vi "Acquisition next state logic_May contain upgrade.vi"(0 "Message Queues":T5, 5 "Acquired z-plane index":i32, 7 "Logging queue element":T1={"Imaging Protocol"=enum."Live Imaging", "Number of Trials"=0, "Frame Size"=512, "# Averaged frames"=0, "Dwell time (us)"=0.0, "Index of Z-plane"=0, "Timelapse?"=FALSE, "Logging process is active"=FALSE, "Speed logging enabled"=FALSE, "tdms file ref"=refnum, "path"=path "", "Trial Number"=0, "Expected # points acquired"=FALSE, "Manually stopped"=FALSE, "Last trial"=FALSE, "Ch0 data"=[], "Ch1 data"=[], "Ref Data"=[], "Ref Frame Time"=[], "Image Time"=[], "Continuous Time"=[], "Ref X Length"=0, "Ref Y Length"=0, "# Ref Averaged frames"=0, "Ref Dwell time (us)"=0.0, "Points acquired"={"Ch0 last trial"=0, "Ch1 last trial"=0, "All trials"=0}, "HW Timings File"=refnum} {"Ref Dwell time (us)" format="%#.6g"; "Frame Size" items=["100X100"=100, "128X128"=128, "200X200"=200, "256X256"=256, "512X512"=512, "1024x1024"=1024, "2048x2048"=2048]; "Dwell time (us)" format="%#.6g"}, 9 "Imaging Protocol":T2=enum."Live Imaging", 11 "error in":errorcluster) -> (6 "Index of next Z-plane to acquire":i32, 15 "error out":errorcluster)   [LabVIEW 2020]
uses:
  User Interface/Queue/Message Queue/Typedefs/All Message Queues.ctl
  User Interface/Queue/Message Queue/Typedefs/Message Cluster.ctl
  Typedefs/Logging queue element.ctl
  Typedefs/Imaging Protocols enum.ctl
  Typedefs/Frame Size.ctl
  Typedefs/Acquired points count.ctl
  Typedefs/Read Write Enum.ctl
  Global Variables/General Globals.vi
  Typedefs/Top level VI states.ctl
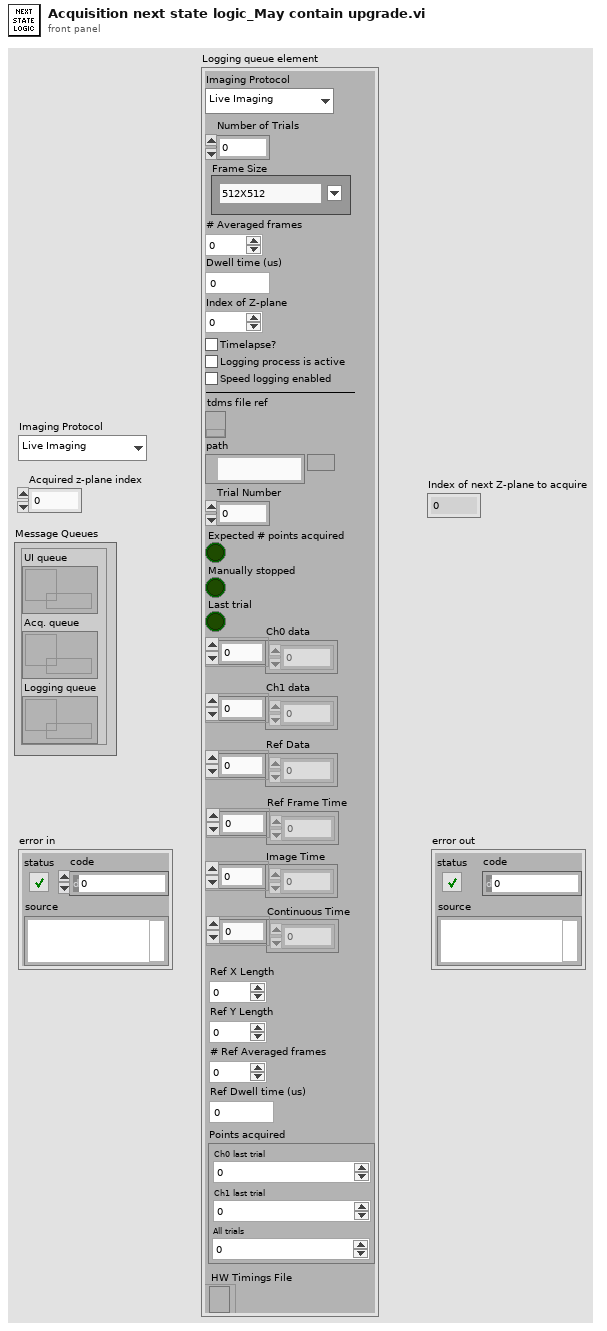
[diagram p1: front panel]
types:
  T1 = typedef "Logging queue element.ctl" = cluster{"Imaging Protocol":T2, "Number of Trials":u16, "Frame Size":T3, "# Averaged frames":u16, "Dwell time (us)":dbl, "Index of Z-plane":i32, "Timelapse?":bool, "Logging process is active":bool, "Speed logging enabled":bool, "tdms file ref":refnum<k34>, "path":path, "Trial Number":i32, "Expected # points acquired":bool, "Manually stopped":bool, "Last trial":bool, "Ch0 data":u32[], "Ch1 data":u32[], "Ref Data":u32[], "Ref Frame Time":u64[], "Image Time":u64[], "Continuous Time":u64[], "Ref X Length":u16, "Ref Y Length":u16, "# Ref Averaged frames":u16, "Ref Dwell time (us)":dbl, "Points acquired":T4, "HW Timings File":refnum<file>}
  T2 = typedef "Imaging Protocols enum.ctl" = enum16{"AOL Z-Stack", "Motor Z Stack", "Functional Acquisition", "Single Plane Acquisition", "Volume Acquisition", "Live Imaging", "Live Plane Imaging", "Live Volume Imaging"}
  T3 = typedef "Frame Size.ctl" = u16
  T4 = typedef "Acquired points count.ctl" = cluster{"Ch0 last trial":u64, "Ch1 last trial":u64, "All trials":u64}
  T5 = typedef "All Message Queues.ctl" = cluster{"UI queue":refnum<queue>, "Acq. queue":refnum<queue>, "Logging queue":refnum<queue>}
  T6 = typedef "Read Write Enum.ctl" = enum16{"Read", "Write"}
  T7 = typedef "Top level VI states.ctl" = enum16{"None", "Initialise UI", "<STACK PROTOCOL STATES>", "AOL Zstack-START", "AOL Zstack-STOP", "Motor Zstack-START", "Motor Zstack-STOP", "<ACQUISITION PROTOCOL STATES> ", "Functional Acquisition-START", "Functional Acquisition-STOP", "Single Plane Acquisition-START", "Single Plane Acquisition-STOP", "Volume Acquisition-START", "Volume Acquisition-STOP", "<LIVE IMAGING PROTOCOL STATES>", "Live Imaging-START", "Live Imaging-STOP", "Live Plane Imaging-START", "Live Plane Imaging-STOP", "Live Volume Imaging-START", "Live Volume Imaging-STOP", "<MOVEMENT CORRECTION PROTOCOL STATES>", "EXIT"}
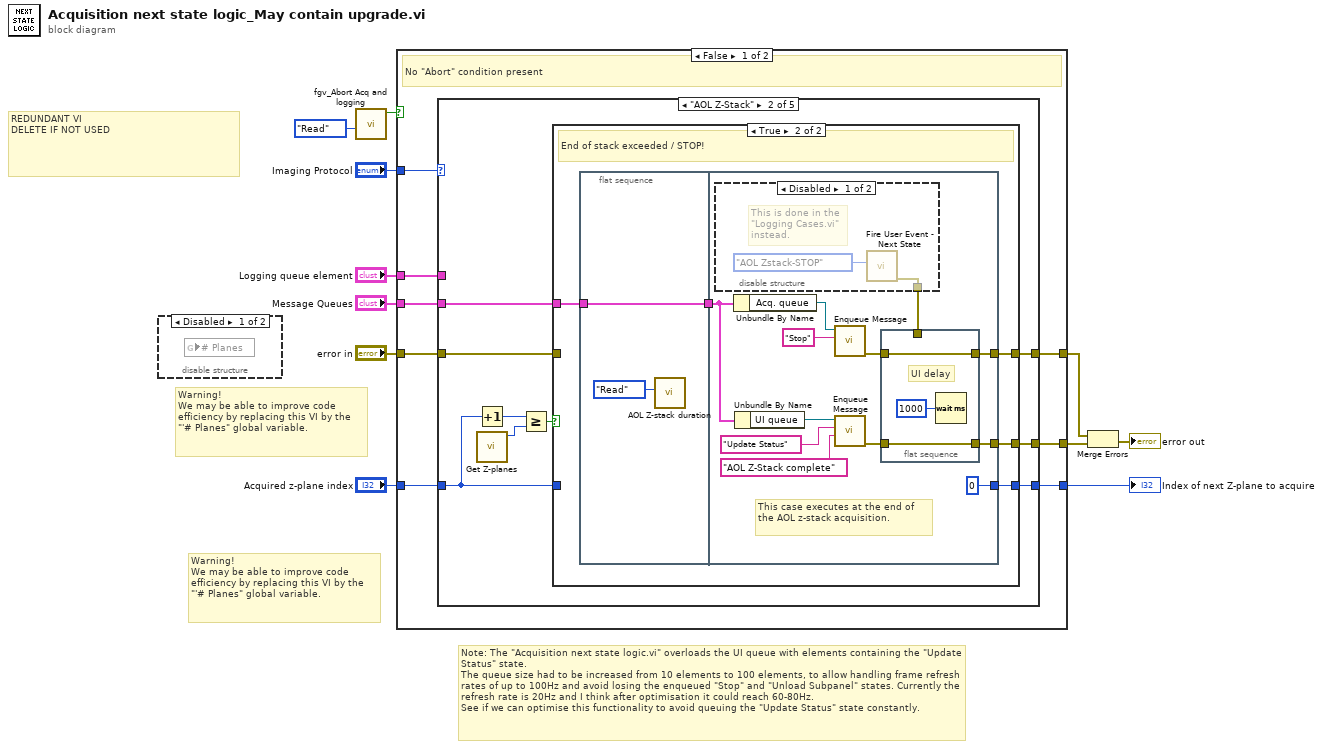
[diagram p0: block diagram]
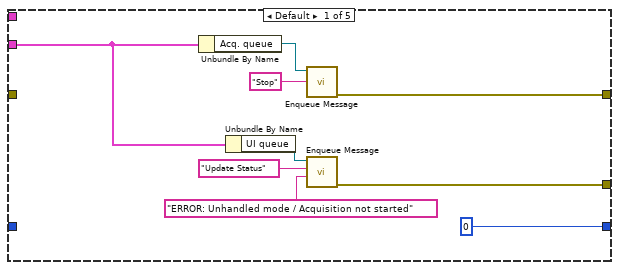
[diagram p3: hidden frame]
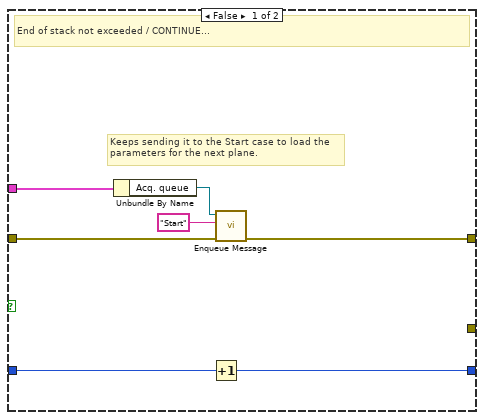
[diagram p4: hidden frame]
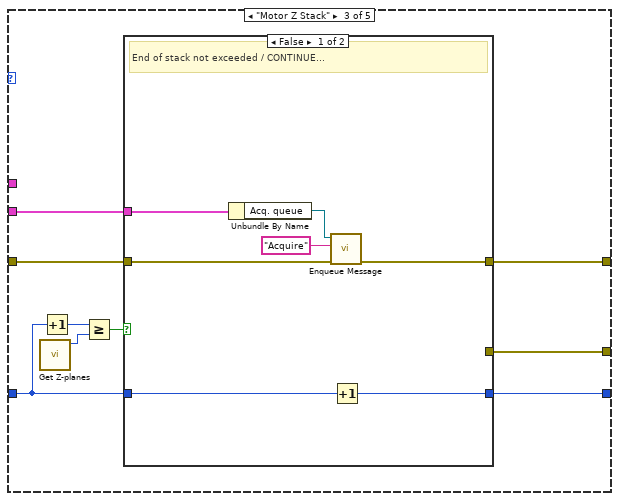
[diagram p6: hidden frame]
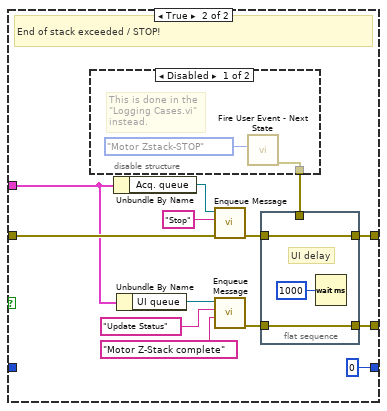
[diagram p7: hidden frame]
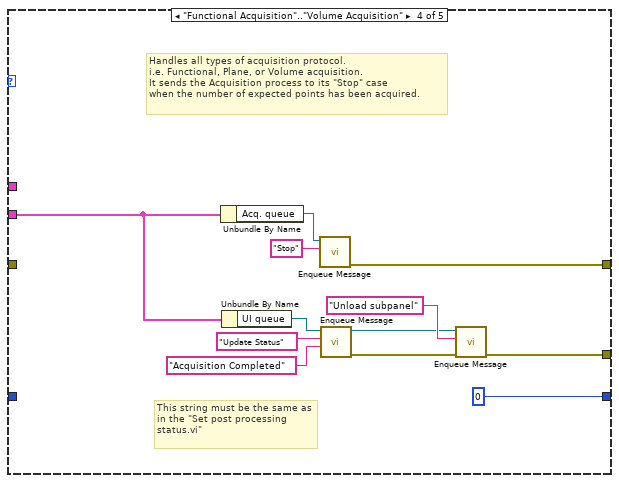
[diagram p9: hidden frame]
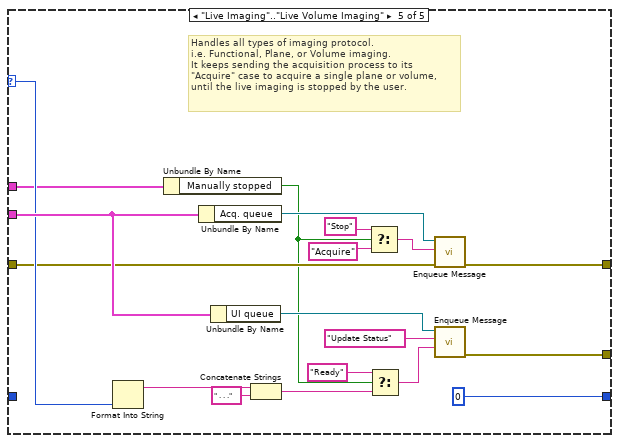
[diagram p10: hidden frame]
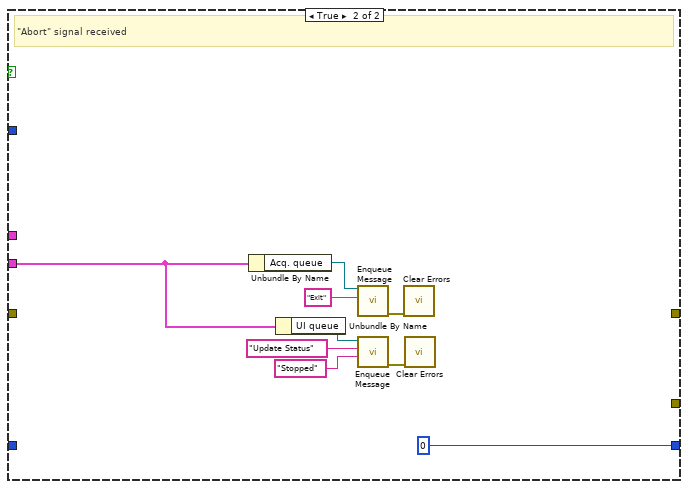
[diagram p11: hidden frame]
diagram:
  # "REDUNDANT VI\nDELETE IF NOT USED"
  # "Note: The \"Acquisition next state logic.vi\" overloads the UI queue with elements containing the \"Update Status\" state.\nThe queue size had to be increased from 10 elements to 100 elements, to allow handling frame refresh rates of up to 100Hz and avoid losing the enqueued \"Stop\" and \"Unload Subpanel\" states. Currently the refresh rate is 20Hz and I think after optimisation it could reach 60-80Hz.\nSee if we can optimise this functionality to avoid queuing the \"Update Status\" state constantly."
  # "Warning!\nWe may be able to improve code efficiency by replacing this VI by the \"'# Planes\" global variable."
  # "Warning!\nWe may be able to improve code efficiency by replacing this VI by the \"'# Planes\" global variable."
  n1 = disable-structure "Diagram Disable Structure" shown="Disabled" {
    frame Disabled {
      n2 = global read "General Globals.vi" "# Planes"() -> ()  [unwired: 1 in]
    }
    frame Enabled {
    }
  }
  n3 = call "fgv_Abort Acq and logging.vi"("Function"=Read_Write_Enum."Read") -> ("Abort acquisition"=w1:bool)  [unwired: 9 in, 1 out]
  n4 = case shown="False" w1 {
    tunnel: [w19 _] -> w6
    tunnel: "error in" -> [w18 _]
    tunnel: [w17 0] -> w8
    tunnel: [w16 _] -> w5
    tunnel: "Acquired z-plane index" -> [w15 _]
    tunnel: "Imaging Protocol" -> [w13 _]
    tunnel: "Message Queues" -> [w14 w136]
    tunnel: "Logging queue element" -> [w12 _]
    frame False {
      # "No \"Abort\" condition present"
      n5 = case shown="\"AOL Z-Stack\"" w13 {
        selector: w13 -> [_ _ _ _ w127]
        tunnel: w18 -> [_ w32 w76 _ w124]
        tunnel: [w27 w36 w77 w113 w133] -> w19
        tunnel: [0 w34 w75 0 0] -> w17
        tunnel: w15 -> [_ w33 w70 _ _]
        tunnel: [w24 w35 w74 w105 w131] -> w16
        tunnel: w14 -> [w21 w31 w73 w109 w128]
        tunnel: w12 -> [_ _ _ _ w123]
        frame Default {
          n6 = Unbundle By Name(w21) -> ("Acq. queue"=w22:refnum<queue>)
          n7 = Unbundle By Name(w21) -> ("UI queue"=w23:refnum<queue>)
          n8 = call "Enqueue Message.vi"("Message"="Stop", "Queue"=w22) -> ("error out"=w27:errorcluster)  [unwired: 8 in, 1 out]
          n9 = call "Enqueue Message.vi"("Message Data"="ERROR: Unhandled mode / Acquisition not started" ("Message"), "Message"="Update Status", "Queue"=w23) -> ("error out"=w24:errorcluster)  [unwired: 7 in, 1 out]
        }
        frame "AOL Z-Stack" {
          n10 = Increment(x=w33) -> (x+1=w29:i32)
          n11 = call "Get Z-planes.vi"() -> ("# of Z-planes"=w37:i32)  [unwired: 7 in, 4 out]
          n12 = Greater Or Equal?(x=w29, y=w37) -> (x >= y?=w30:bool)
          n13 = case shown="True" w30 {
            tunnel: [w43 w47] -> w36
            tunnel: w32 -> [w42 _]
            tunnel: w33 -> [w41 _]
            tunnel: [w38 w49] -> w34
            tunnel: [_ w46] -> w35
            tunnel: w31 -> [w39 w48]
            frame False {
              # "Keeps sending it to the Start case to load the\nparameters for the next plane."
              # "End of stack not exceeded / CONTINUE..."
              n14 = Unbundle By Name(w39) -> ("Acq. queue"=w40:refnum<queue>)
              n15 = Increment(x=w41) -> (x+1=w38:i32)
              n16 = call "Enqueue Message.vi"("error in (no error)"=w42, "Message"="Start", "Queue"=w40) -> ("error out"=w43:errorcluster)  [unwired: 7 in, 1 out]
            }
            frame True {
              # "End of stack exceeded / STOP!"
              n17 = flat-sequence {
                tunnel: w48 -> [w51]
                tunnel: [w51] -> w45
                tunnel: [0] -> w49
                tunnel: [w55] -> w47
                tunnel: [w53] -> w46
                tunnel: w45 -> [w60]
                frame #0 {
                  n18 = call "AOL Z-stack duration.vi"("Function"=Read_Write_Enum."Read") -> ()  [unwired: 10 in, 1 out]
                }
                frame #1 {
                  # "This case executes at the end of the AOL z-stack acquisition."
                  n19 = disable-structure shown="Disabled" {
                    disable-tunnel: [w64 _] -> w52
                    frame Disabled {
                      # "This is done in the \"Logging Cases.vi\" instead."
                      n20 = call "Fire User Event - Next State.vi"("\"UI Handler loop\" case to execute"=Top_level_VI_states."AOL Zstack-STOP" ("event data / imaging mode")) -> ("Error Out"=w64:errorcluster)  [unwired: 10 in]
                    }
                    frame Enabled {
                    }
                  }
                  n21 = Unbundle By Name(w60) -> ("Acq. queue"=w61:refnum<queue>)
                  n22 = Unbundle By Name(w60) -> ("UI queue"=w59:refnum<queue>)
                  n23 = call "Enqueue Message.vi"("Message"="Stop", "Queue"=w61) -> ("error out"=w56:errorcluster)  [unwired: 8 in, 1 out]
                  n24 = call "Enqueue Message.vi"("Message Data"="AOL Z-Stack complete" ("Message"), "Message"="Update Status", "Queue"=w59) -> ("error out"=w54:errorcluster)  [unwired: 7 in, 1 out]
                  n25 = flat-sequence {
                    tunnel: w56 -> [w67]
                    tunnel: [w67] -> w55
                    tunnel: w54 -> [w66]
                    tunnel: [w66] -> w53
                    tunnel: w52 -> [_]
                    frame #0 {
                      # "UI delay"
                      n26 = Wait (ms)(milliseconds to wait=u32 1000) -> ()  [unwired: 1 out]
                    }
                  }
                }
              }
            }
          }
        }
        frame "Motor Z Stack" {
          n27 = call "Get Z-planes.vi"() -> ("# of Z-planes"=w72:i32)  [unwired: 7 in, 4 out]
          n28 = Increment(x=w70) -> (x+1=w69:i32)
          n29 = Greater Or Equal?(x=w69, y=w72) -> (x >= y?=w71:bool)
          n30 = case shown="False" w71 {
            tunnel: [w83 w88] -> w77
            tunnel: w76 -> [w82 w95]
            tunnel: w70 -> [w81 _]
            tunnel: [w78 0] -> w75
            tunnel: [_ w86] -> w74
            tunnel: w73 -> [w79 w93]
            frame False {
              # "End of stack not exceeded / CONTINUE..."
              n31 = Unbundle By Name(w79) -> ("Acq. queue"=w80:refnum<queue>)
              n32 = call "Enqueue Message.vi"("error in (no error)"=w82, "Message"="Acquire", "Queue"=w80) -> ("error out"=w83:errorcluster)  [unwired: 7 in, 1 out]
              n33 = Increment(x=w81) -> (x+1=w78:i32)
            }
            frame True {
              # "End of stack exceeded / STOP!"
              n34 = disable-structure shown="Disabled" {
                disable-tunnel: [w98 _] -> w85
                frame Disabled {
                  # "This is done in the \"Logging Cases.vi\" instead."
                  n35 = call "Fire User Event - Next State.vi"("\"UI Handler loop\" case to execute"=Top_level_VI_states."Motor Zstack-STOP" ("event data / imaging mode")) -> ("Error Out"=w98:errorcluster)  [unwired: 10 in]
                }
                frame Enabled {
                }
              }
              n36 = Unbundle By Name(w93) -> ("Acq. queue"=w94:refnum<queue>)
              n37 = Unbundle By Name(w93) -> ("UI queue"=w92:refnum<queue>)
              n38 = call "Enqueue Message.vi"("error in (no error)"=w95, "Message"="Stop", "Queue"=w94) -> ("error out"=w89:errorcluster)  [unwired: 7 in, 1 out]
              n39 = call "Enqueue Message.vi"("Message Data"="Motor Z-Stack complete" ("Message"), "Message"="Update Status", "Queue"=w92) -> ("error out"=w87:errorcluster)  [unwired: 7 in, 1 out]
              n40 = flat-sequence {
                tunnel: w89 -> [w101]
                tunnel: [w101] -> w88
                tunnel: w87 -> [w100]
                tunnel: [w100] -> w86
                tunnel: w85 -> [_]
                frame #0 {
                  # "UI delay"
                  n41 = Wait (ms)(milliseconds to wait=u32 1000) -> ()  [unwired: 1 out]
                }
              }
            }
          }
        }
        frame "Functional Acquisition".."Volume Acquisition" {
          # "This string must be the same as in the \"Set post processing status.vi\""
          # "Handles all types of acquisition protocol.\ni.e. Functional, Plane, or Volume acquisition.\nIt sends the Acquisition process to its \"Stop\" case\nwhen the number of expected points has been acquired."
          n42 = Unbundle By Name(w109) -> ("Acq. queue"=w110:refnum<queue>)
          n43 = Unbundle By Name(w109) -> ("UI queue"=w108:refnum<queue>)
          n44 = call "Enqueue Message.vi"("Message"="Stop", "Queue"=w110) -> ("error out"=w113:errorcluster)  [unwired: 8 in, 1 out]
          n45 = call "Enqueue Message.vi"("Message Data"="Acquisition Completed" ("Message"), "Message"="Update Status", "Queue"=w108) -> ("error out"=w106:errorcluster, "Queue out"=w104:refnum<queue>)  [unwired: 7 in]
          n46 = call "Enqueue Message.vi"("error in (no error)"=w106, "Message"="Unload subpanel", "Queue"=w104) -> ("error out"=w105:errorcluster)  [unwired: 7 in, 1 out]
        }
        frame "Live Imaging".."Live Volume Imaging" {
          # "Handles all types of imaging protocol.\ni.e. Functional, Plane, or Volume imaging.\nIt keeps sending the acquisition process to its\n\"Acquire\" case to acquire a single plane or volume,\nuntil the live imaging is stopped by the user."
          n47 = Format Into String(w127) -> (resulting string=w126:string)  [unwired: 3 in, 1 out]
          n48 = Unbundle By Name(w123) -> ("Manually stopped"=w116:bool)
          n49 = Unbundle By Name(w128) -> ("Acq. queue"=w129:refnum<queue>)
          n50 = Unbundle By Name(w128) -> ("UI queue"=w130:refnum<queue>)
          n51 = Concatenate Strings(w126, " . . ." ("string")) -> (w119:string)
          n52 = Select(t="Stop" ("Message"), s=w116, f="Acquire" ("Message")) -> (s? t:f=w120:string)
          n53 = Select(t="Ready", s=w116, f=w119) -> (s? t:f=w118:string)
          n54 = call "Enqueue Message.vi"("error in (no error)"=w124, "Message"=w120, "Queue"=w129) -> ("error out"=w133:errorcluster)  [unwired: 7 in, 1 out]
          n55 = call "Enqueue Message.vi"("Message Data"=w118, "Message"="Update Status", "Queue"=w130) -> ("error out"=w131:errorcluster)  [unwired: 7 in, 1 out]
        }
      }
    }
    frame True {
      # "\"Abort\" signal received"
      n56 = Unbundle By Name(w136) -> ("Acq. queue"=w140:refnum<queue>)
      n57 = Unbundle By Name(w136) -> ("UI queue"=w137:refnum<queue>)
      n58 = call "Enqueue Message.vi"("Message"="Exit", "Queue"=w140) -> ("error out"=w134:errorcluster)  [unwired: 8 in, 1 out]
      n59 = call "Enqueue Message.vi"("Message Data"="Stopped" ("Message"), "Message"="Update Status", "Queue"=w137) -> ("error out"=w135:errorcluster)  [unwired: 7 in, 1 out]
      n60 = call <vilib>:"Clear Errors.vi"("error in (no error)"=w134) -> ()  [unwired: 5 in, 2 out]
      n61 = call <vilib>:"Clear Errors.vi"("error in (no error)"=w135) -> ()  [unwired: 5 in, 2 out]
    }
  }
  "Index of next Z-plane to acquire" <- w8
  n62 = Merge Errors(w6, w5) -> (→"error out":errorcluster)
